vi "PC_PING.vi"() -> ()   [LabVIEW 2013]
uses:
  Controls/PingQueueTypDef.ctl
  Controls/stopQue.ctl
panel:
  out "stop":bool
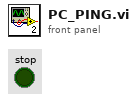
[diagram p1: front panel]
types:
  T1 = typedef "stopQue.ctl" = cluster{"stop":bool}
  T2 = typedef "PingQueueTypDef.ctl" = cluster{"Computers not on":string[]}
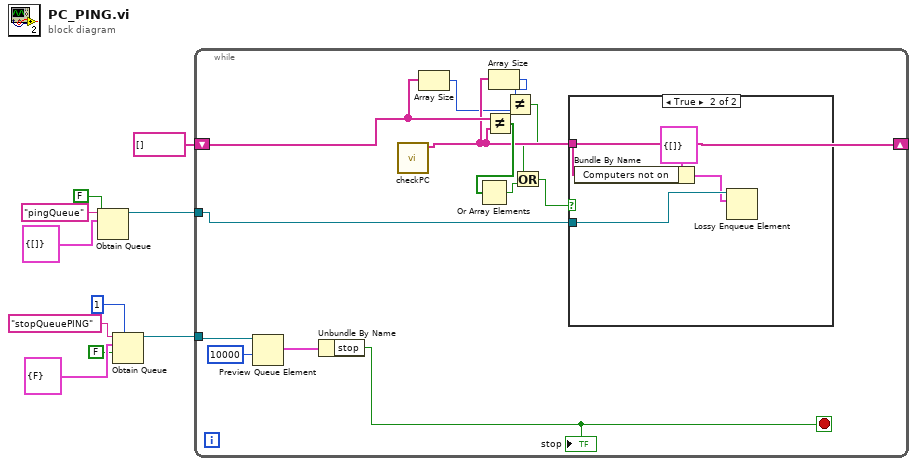
[diagram p0: block diagram]
diagram:
  n1 = Obtain Queue(name (unnamed)="pingQueue", element data type=T2 {"Computers not on"=[]}, create if not found? (T)=FALSE) -> (queue out=w7:refnum<queue>)  [unwired: 2 in, 2 out]
  n2 = Obtain Queue(max queue size (-1, unlimited)=1, name (unnamed)="stopQueuePING", element data type=T1 {"stop"=FALSE}, create if not found? (T)=FALSE) -> (queue out=w1:refnum<queue>)  [unwired: 1 in, 2 out]
  n3 = while {
    shift-right: [w16] -> _
    shift-left: string[] [] ("Computers not on") -> [w17]
    tunnel: w7 -> [w22]
    tunnel: w1 -> [w21]
    stop <- w19 stop-if-true
    n4 = Preview Queue Element(queue=w21, timeout in ms (-1)=10000) -> (element=w20:T1)  [unwired: 1 in, 3 out]
    n5 = Unbundle By Name(w20) -> ("stop"=w19:bool)
    "stop" <- w19
    n6 = call "checkPC.vi"() -> ("Computers not on"=w16:string[])  [unwired: 9 in, 2 out]
    n7 = Array Size(array=w17) -> (size(s)=w14:i32)
    n8 = Not Equal?(x=w17, y=w16) -> (x != y?=w23:bool[])
    n9 = Or Array Elements(Boolean array=w23) -> (logical OR=w13:bool)
    n10 = Array Size(array=w16) -> (size(s)=w15:i32)
    n11 = Not Equal?(x=w15, y=w14) -> (x != y?=w12:bool)
    n12 = Or(x=w12, y=w13) -> (x .or. y?=w11:bool)
    n13 = case shown="True" w11 {
      tunnel: w22 -> [_ w27]
      tunnel: w16 -> [_ w25]
      frame False {
      }
      frame True {
        n14 = Bundle By Name(cluster=T2 {"Computers not on"=[]}, "Computers not on"=w25) -> (w24:T2)
        n15 = Lossy Enqueue Element(queue=w27, element=w24) -> ()  [unwired: 1 in, 4 out]
      }
    }
  }
